vi "loop_display - alternative.vi"(8 "error in":errorcluster, 9 "timing source":string="1 kHz", 11 "reference cluster":T1) -> (0 "error out":errorcluster)   [LabVIEW 2015]
uses:
  Type Definitions/notifier_elements_GUI.ctl
  <vilib>/Platform/TimedLoop/XDataNode/XDataNode.xnode
  <vilib>/Platform/TimedLoop/XDataNode/timing_clust.ctl
  <vilib>/Platform/TimedLoop/XDataNode/XDNodeRunTimeDep.lvlib
  <vilib>/Platform/TimedLoop/XDataNode/wakeup.ctl
  <vilib>/Platform/TimedLoop/XDataNode/nitl_modes.ctl
  Type Definitions/data.ctl
  Type Definitions/control_references.ctl
  Type Definitions/notifier_elements_write.ctl
  Type Definitions/notifier_elements_DAQ.ctl
  Type Definitions/reference_cluster.ctl
  Type Definitions/vars_settings.ctl
  Type Definitions/vars_runtime.ctl
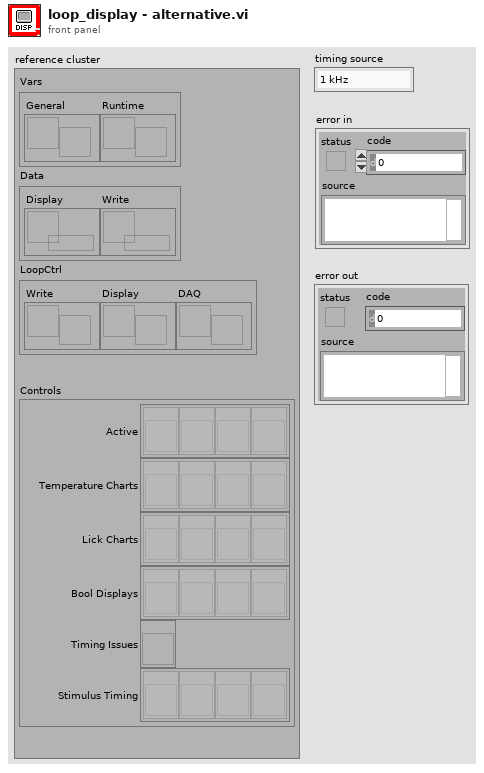
[diagram p1: front panel]
types:
  T1 = typedef "reference_cluster.ctl" = cluster{"Vars":cluster{"General":refnum<notifier>, "Runtime":refnum<notifier>}, "Data":cluster{"Display":refnum<queue>, "Write":refnum<queue>}, "LoopCtrl":cluster{"Write":refnum<notifier>, "Display":refnum<notifier>, "DAQ":refnum<notifier>}, "Controls":T2}
  T2 = typedef "control_references.ctl" = cluster{"Active":refnum<vi>[], "Temperature Charts":refnum<vi>[], "Lick Charts":refnum<vi>[], "Bool Displays":refnum<vi>[], "Timing Issues":refnum<vi>, "Stimulus Timing":refnum<vi>[]}
  T3 = typedef "XDNodeRunTimeDep.lvlib/timing_clust.ctl" = cluster{"Expected End [f-1]":u64, "Actual End [f-1]":u64, "Finished Late? [f-1]":bool, "Expected End [i-1]":u64, "Actual End [i-1]":u64, "Finished Late? [i-1]":bool, "Expected Start [i]":u64, "Actual Start [i]":u64, "Expected Start [f]":u64, "Actual Start [f]":u64, "Source Name":string, "Structure Name":string, "Period":i64, "Deadline":i64, "Offset":i64, "Start":i64, "Priority":i32, "Timeout":i32, "Mode":T4, "Wakeup Reason":T5, "Error":errorcluster, "Source Type":string, "Secondary Source Type":string, "Global End Time":u64, "Global Start Time":u64, "Frame Duration":u64, "Iteration Duration":u64, "Assigned CPU":i32, "I/O Scan Engine Mode":u32}
  T4 = typedef "XDNodeRunTimeDep.lvlib/nitl_modes.ctl" = enum32{"No Change", "Process missed periods, maintain original phase", "Discard missed periods, maintain original phase", "Process missed periods, ignore original phase", "Discard missed periods, ignore original phase"}
  T5 = typedef "XDNodeRunTimeDep.lvlib/wakeup.ctl" = enum32{"Normal", "Aborted", "Asynchronous wakeup", "Timing source error", "Timed loop error", "Timeout"}
  T6 = typedef "notifier_elements_GUI.ctl" = enum16{"GUI - Initialize", "GUI - Pause", "GUI - Run", "GUI - Quit"}
  T7 = typedef "vars_settings.ctl" = cluster{"wait min":u16, "wait max":u16, "d stim":u16, "d timeout":u16, "timeout win":u16, "base temp":sgl, "stim amps":i32[], "active":bool, "pairing":bool, "clean tubes":bool}
  T8 = typedef "data.ctl" = cluster{"time":timestamp, "finished late":bool, "temp out":dbl[], "temp in":dbl[], "lick in":dbl[], "reward":bool[], "lick":bool[], "stim":bool[], "catch":bool[]}
  T9 = typedef "vars_runtime.ctl" = cluster{"wait count t":u16, "stim count t":u16, "stim count n":u16, "n hit":u16, "n catch":u16, "next temp":sgl, "catch":bool, "stimulus":bool, "reward given":bool, "lick":bool, "next reward":bool}
  T10 = cluster{"[0]":bool, "[1]":bool, "[2]":bool, "[3]":bool}
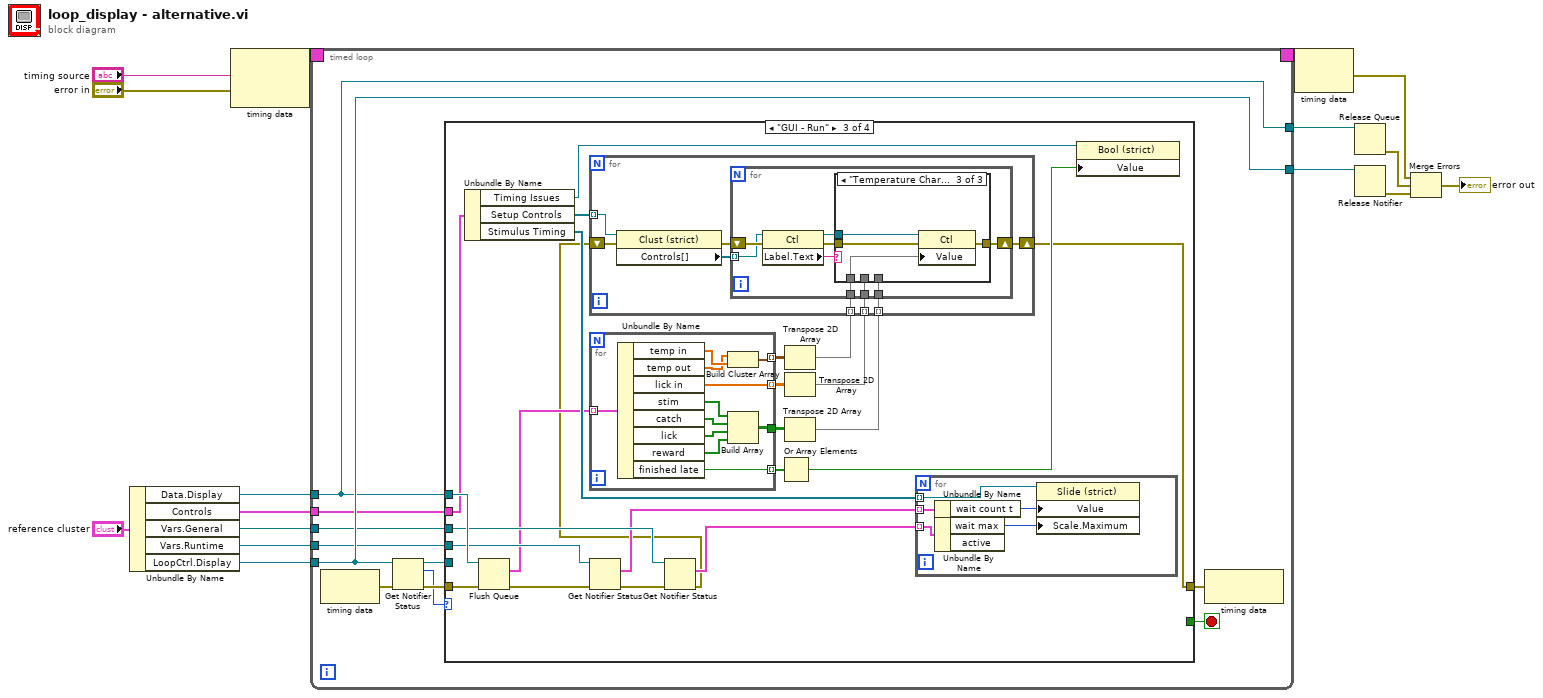
[diagram p0: block diagram]
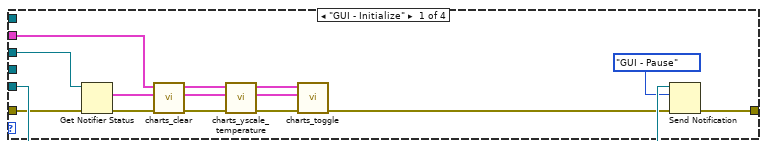
[diagram p2: hidden frame]
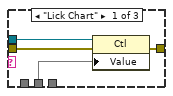
[diagram p4: hidden frame]
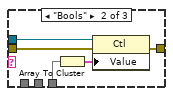
[diagram p5: hidden frame]
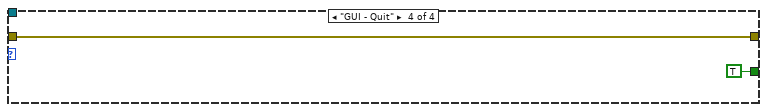
[diagram p6: hidden frame]
diagram:
  n1 = Unbundle By Name("reference cluster") -> ("Data.Display"=w3:refnum<queue>, "Controls"=w4:T2, "Vars.General"=w5:refnum<notifier>, "Vars.Runtime"=w1:refnum<notifier>, "LoopCtrl.Display"=w2:refnum<notifier>)
  n2 = node-c288("timing source", "error in") -> (w16:T3)
  n3 = timed-loop "Display" {
    timing: w16 -> [_]
    timing-out: [_] -> w15
    tunnel: w5 -> [w26]
    tunnel: w4 -> [w25]
    tunnel: [w27] -> w12
    tunnel: [w18] -> w9
    tunnel: w3 -> [w18]
    tunnel: w2 -> [w27]
    tunnel: w1 -> [w17]
    stop <- w24 stop-if-true
    n4 = node-c288() -> (w23:errorcluster)  [unwired: 1 in]
    n5 = Get Notifier Status(notifier=w27, error in (no error)=w23) -> (notifier out=w22:refnum<notifier>, current notification=w20:T6, error out=w21:errorcluster)  [unwired: 2 out]
    n6 = case shown="\"GUI - Run\"" w20 {
      tunnel: w18 -> [_ _ w66 _]
      tunnel: w26 -> [w37 _ w65 _]
      tunnel: [w41 w43 w46 w113] -> w19
      tunnel: w25 -> [w34 _ w64 _]
      tunnel: [_ _ _ TRUE] -> w24
      tunnel: w22 -> [w42 _ _ _]
      tunnel: w21 -> [w38 w43 w61 w113]
      tunnel: w17 -> [_ _ w60 _]
      frame "GUI - Initialize" {
        n7 = Get Notifier Status(notifier=w37, error in (no error)=w38) -> (current notification=w33:T7[], error out=w36:errorcluster)  [unwired: 3 out]
        n8 = call "charts_clear.vi"("error in"=w36, "vars general"=w33, "control cluster"=w34) -> ("error out"=w39:errorcluster, "vars general"=w32:T7[], "control cluster"=w35:T2)  [unwired: 6 in]
        n9 = call "charts_yscale_temperature.vi"("error in"=w39, "vars general"=w32, "control cluster"=w35) -> ("error out"=w31:errorcluster, "vars general"=w30:T7[], "control cluster"=w29:T2)  [unwired: 6 in]
        n10 = call "charts_toggle.vi"("error in (no error)"=w31, "vars general in"=w30, "control cluster in"=w29) -> ("error out"=w28:errorcluster)  [unwired: 6 in, 2 out]
        n11 = Send Notification(notification=notifier_elements_GUI."GUI - Pause", notifier=w42, error in (no error)=w28) -> (error out=w41:errorcluster)  [unwired: 1 out]
      }
      frame "GUI - Pause" {
      }
      frame "GUI - Run" {
        n12 = Unbundle By Name(w64) -> ("Timing Issues"=w56:refnum<vi>, "Setup Controls"=w55:refnum<vi>[], "Stimulus Timing"=w54:refnum<vi>[])
        n13 = Flush Queue(queue=w66, error in (no error)=w61) -> (remaining elements=w53:T8[], error out=w58:errorcluster)  [unwired: 1 out]
        n14 = for {
          tunnel: w53 -> [w73] mode=indexing
          tunnel: [w72] -> w52 mode=indexing
          tunnel: [w71] -> w50 mode=indexing
          tunnel: [w70] -> w45
          tunnel: [w69] -> w48 mode=indexing
          n15 = Unbundle By Name(w73) -> ("temp in"=w68:dbl[], "temp out"=w67:dbl[], "lick in"=w71:dbl[], "stim"=w77:bool[], "catch"=w75:bool[], "lick"=w74:bool[], "reward"=w76:bool[], "finished late"=w69:bool)
          n16 = Build Cluster Array(w67, w68) -> (w72:cluster{"temp in":dbl, "temp in":dbl}[])
          n17 = Build Array(w77, w75, w74, w76) -> (w70:bool[][])
        }
        n18 = Get Notifier Status(notifier=w60, error in (no error)=w58) -> (current notification=w57:T9[], error out=w59:errorcluster)  [unwired: 3 out]
        n19 = Get Notifier Status(notifier=w65, error in (no error)=w59) -> (current notification=w62:T7[], error out=w47:errorcluster)  [unwired: 3 out]
        n20 = Or Array Elements(Boolean array=w48) -> (logical OR=w63:bool)
        n21 = Transpose 2D Array(2D array=w52) -> (transposed array=w51:cluster{"temp in":dbl, "temp in":dbl}[][])
        n22 = Transpose 2D Array(2D array=w50) -> (transposed array=w49:dbl[][])
        n23 = Transpose 2D Array(2D array=w45) -> (transposed array=w44:bool[][])
        n24 = for {
          tunnel: w55 -> [w90] mode=indexing
          tunnel: w51 -> [w83] mode=indexing
          tunnel: w49 -> [w89] mode=indexing
          shift-right: [w86] -> w46
          shift-left: w47 -> [w88]
          tunnel: w44 -> [w84] mode=indexing
          n25 = property class="Clust (strict)"(reference=w90, error in=w88) -> (error out=w87:errorcluster, "Controls[]"=w85:refnum<vi>[])  [unwired: 1 out]
          n26 = for {
            tunnel: w83 -> [w99]
            tunnel: w89 -> [w98]
            shift-right: [w93] -> w86
            shift-left: w87 -> [w94]
            tunnel: w85 -> [w92] mode=indexing
            tunnel: w84 -> [w91]
            n27 = property class="Ctl"(reference=w92, error in=w94) -> (reference out=w97:refnum<vi>, error out=w96:errorcluster, "Label.Text"=w95:string)
            n28 = case shown="\"Temperature Chart\", Default" w95 {
              tunnel: w99 -> [_ _ w109]
              tunnel: w98 -> [w100 _ _]
              tunnel: w97 -> [w103 w107 w112]
              tunnel: w96 -> [w102 w106 w111]
              tunnel: [w101 w108 w110] -> w93
              tunnel: w91 -> [_ w104 _]
              frame "Lick Chart" {
                n29 = property class="Ctl"(reference=w103, error in=w102, "Value"=w100) -> (error out=w101:errorcluster)  [unwired: 1 out]
              }
              frame "Bools" {
                n30 = Array To Cluster(array=w104) -> (cluster=w105:T10)
                n31 = property class="Ctl"(reference=w107, error in=w106, "Value"=w105) -> (error out=w108:errorcluster)  [unwired: 1 out]
              }
              frame "Temperature Chart", Default {
                n32 = property class="Ctl"(reference=w112, error in=w111, "Value"=w109) -> (error out=w110:errorcluster)  [unwired: 1 out]
              }
            }
          }
        }
        n33 = for {
          tunnel: w62 -> [w82] mode=indexing
          tunnel: w54 -> [w81] mode=indexing
          tunnel: w57 -> [w79] mode=indexing
          n34 = Unbundle By Name(w79) -> ("wait count t"=w78:u16)
          n35 = Unbundle By Name(w82) -> ("wait max"=w80:u16)  [unwired: 1 out]
          n36 = property class="Slide (strict)"(reference=w81, "Value"=w78, "Scale.Maximum"=w80) -> ()  [unwired: 1 in, 2 out]
        }
        n37 = property on="Property Node" class="Bool (strict)"(reference=w56, "Value"=w63) -> ()  [unwired: 1 in, 2 out]
      }
      frame "GUI - Quit" {
      }
    }
    n38 = node-c288(w19) -> ()  [unwired: 1 out]
  }
  n39 = node-c288(w15) -> (w8:errorcluster)
  n40 = Release Queue(queue=w9) -> (error out=w7:errorcluster)  [unwired: 2 in, 2 out]
  n41 = Release Notifier(notifier=w12) -> (error out=w11:errorcluster)  [unwired: 2 in, 2 out]
  n42 = Merge Errors(w8, w7, w11) -> (→"error out":errorcluster)
